vi "Read File.vi"(8 "error in (no error)":errorcluster, 10 "Path in":path, 11 "Section File Interface":refnum<class "Section File Interface.lvclass">) -> (0 "error out":errorcluster, 2 "SysDef":T1 {"Tree"."Properties"."Type" items=["K_STRING", "K_BOOL", "K_I32", "K_U32", "K_DOUBLE", "K_U64", "K_VARIANT", "K_DEPENDENTFILE", "K_DEPENDENTNODE", "K_DATASOURCENODE", "K_U16", "K_DBLARR", "K_U32ARR", "K_I32ARR", "K_STRINGARR", "K_DICTIONARY", "K_DICTIONARYARR"]})   [LabVIEW 2024, in "ImportExport.lvlib" / "Section File Interface.lvclass"]
uses:
  Section File Interface.lvclass
  <vilib>/NI/NI VeriStand Advanced SysDef API/_Types/SysDef.Export.ctl
  <vilib>/NI/NI VeriStand Advanced SysDef API/_Types/TreeItem.ctl
  <vilib>/NI/NI VeriStand Advanced SysDef API/_Types/TreeItem.Info.ctl
  <vilib>/NI VeriStand/Custom Device API/Custom Device Channel.ctl
  <vilib>/NI VeriStand/Custom Device API/Custom Device Channel Type.ctl
  <vilib>/NI VeriStand/Custom Device API/Custom Device Waveform.ctl
  <vilib>/NI VeriStand/Custom Device API/Custom Device Waveform DataType.ctl
  <vilib>/NI/NI VeriStand Advanced SysDef API/_Types/TreeItem.Property.ctl
  <vilib>/NI/NI VeriStand Advanced SysDef API/_Types/File.DataType.ctl
  advanced-sysdef-api/Source/_Types/SysDef.Export.subSection.ctl
  <vilib>/NI/NI VeriStand Advanced SysDef API/SysDef API/Advanced System Definition.lvlib
  <vilib>/NI VeriStand/Custom Device API/Custom Device API.lvlib
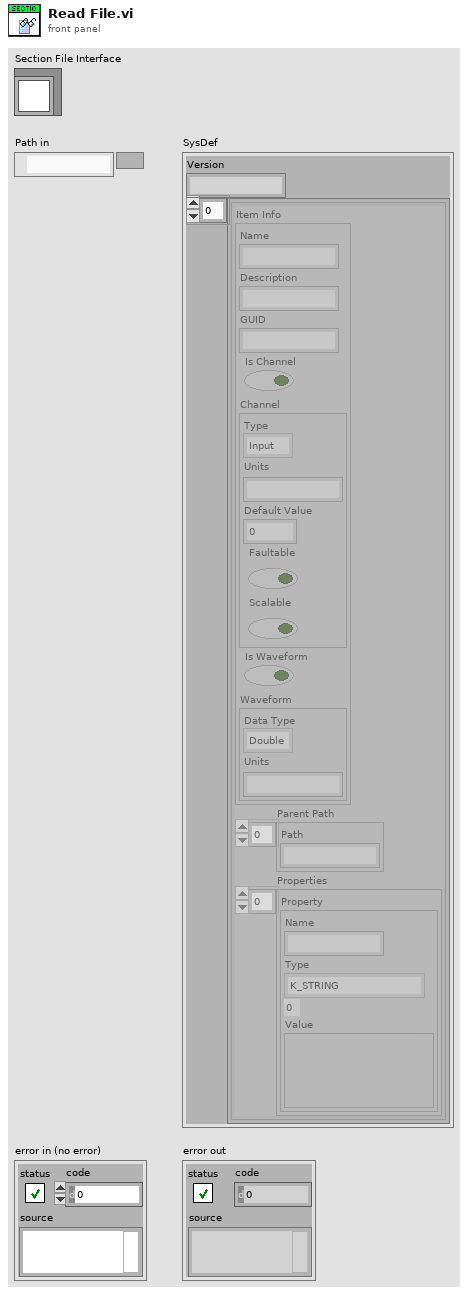
[diagram p1: front panel]
types:
  T1 = typedef "Advanced System Definition.lvlib/SysDef.Export.ctl" = cluster{"Version":string, "Tree":T2[]}
  T2 = typedef "Advanced System Definition.lvlib/TreeItem.ctl" = cluster{"Item Info":T3, "Parent Path":string[], "Properties":T8[]}
  T3 = typedef "Advanced System Definition.lvlib/TreeItem.Info.ctl" = cluster{"Name":string, "Description":string, "GUID":string, "Is Channel":bool, "Channel":T4, "Is Waveform":bool, "Waveform":T6}
  T4 = typedef "Custom Device API.lvlib/Custom Device Channel.ctl" = cluster{"Type":T5, "Units":string, "Default Value":dbl, "Faultable":bool, "Scalable":bool}
  T5 = typedef "Custom Device API.lvlib/Custom Device Channel Type.ctl" = enum16{"Input", "Output"}
  T6 = typedef "Custom Device API.lvlib/Custom Device Waveform.ctl" = cluster{"Data Type":T7, "Units":string}
  T7 = typedef "Custom Device API.lvlib/Custom Device Waveform DataType.ctl" = enum16{"Double", "Complex Double"}
  T8 = typedef "Advanced System Definition.lvlib/TreeItem.Property.ctl" = cluster{"Name":string, "Type":i32, "Value":variant}
  T9 = enum16{"open", "replace", "create", "open or create", "replace or create", "replace or create with confirmation"}
  T10 = typedef "Advanced System Definition.lvlib/SysDef.Export.subSection.ctl" = cluster{"Version":string, "Tree":T2[], "TypeGUID ":string, "ExportedRootNodePath":string}
  T11 = typedef "Advanced System Definition.lvlib/File.DataType.ctl" = cluster{"Version":string, "Data":variant}
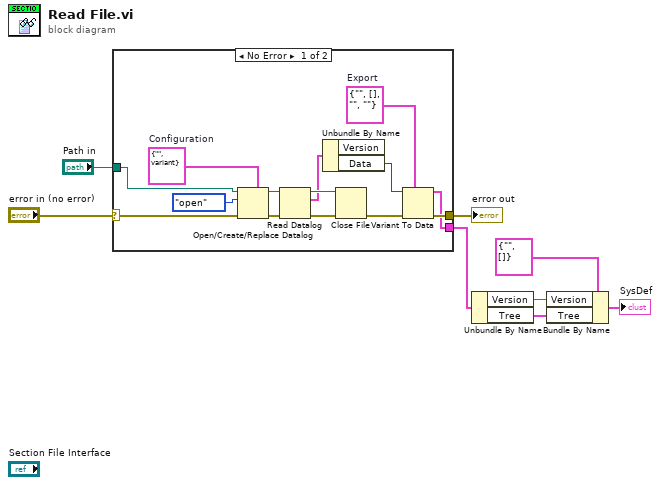
[diagram p0: block diagram]
diagram:
  n1 = case shown="No Error" "error in (no error)" {
    selector: "error in (no error)" -> [w16 w23]
    tunnel: [w10 w23] -> w7
    tunnel: "Path in" -> [w15 _]
    tunnel: [w9 _] -> w3
    frame No Error {
      w13 = T10 {"Version"="", "Tree"=[], "TypeGUID "="", "ExportedRootNodePath"=""}  # Export
      w14 = T11 {"Version"="", "Data"=variant}  # Configuration
      n2 = Open/Create/Replace Datalog(5:w14, 8:w16, 10:T9."open" ("operation (0:open)"), 11:w15) -> (0:w21:errorcluster, 3:w20:refnum<k1>)  [unwired: 2 in, 1 out]
      n3 = Read Datalog(4:w21, 7:w20) -> (0:w19:errorcluster, 2:w17:T11, 3:w18:refnum<k1>)  [unwired: 1 in]
      n4 = Unbundle By Name(w17) -> ("Data"=w12:variant)  [unwired: 1 out]
      n5 = Close File(refnum=w18, error in=w19) -> (error out=w11:errorcluster)  [unwired: 1 out]
      n6 = Variant To Data(error in=w11, type=w13, Variant=w12) -> (data=w9:T10, error out=w10:errorcluster)
    }
    frame Error {
    }
  }
  "error out" <- w7
  n7 = Unbundle By Name(w3) -> ("Version"=w2:string, "Tree"=w1:T2[])
  n8 = Bundle By Name(cluster=T1 {"Version"="", "Tree"=[]} ("SysDef"), "Version"=w2, "Tree"=w1) -> (→"SysDef":T1)
